vi "_Switch Polarity.vi"(0 "Lenses":T1[](array[typedef]), 1 "Start Value":dbl, 2 "Stop Value":dbl, 3 "index":i32, 4 "Unit":bool) -> (5 "Lenses 2":T1[](array[typedef]), 6 "Start Value 2":dbl, 7 "Stop Value 2":dbl)   [LabVIEW 2012]
uses:
  Type/_Lens Property.ctl
  _Global Configuration.vi
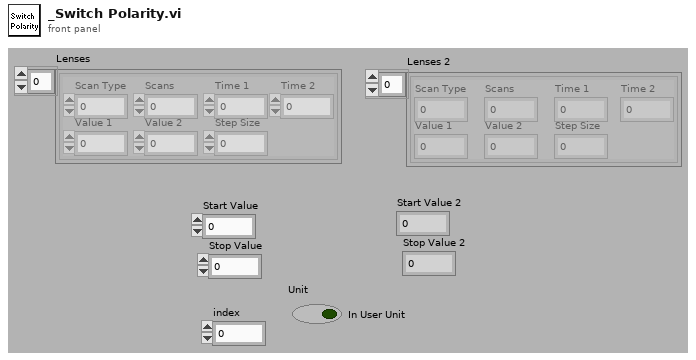
[diagram p1: front panel]
types:
  T1 = typedef "_Lens Property.ctl" = cluster{"Scan Type":u8, "Scans":i32, "Time 1":dbl, "Time 2":dbl, "Value 1":dbl, "Value 2":dbl, "Step Size":dbl}
  T2 = typedef "_RT Instrument 2.ctl" = cluster{"Table":T3[], "Instrument":string[]}
  T3 = typedef "_RT Configuration 2.ctl" = cluster{"Name":string, "Ch#":u8, "Min":dbl, "Max":dbl, "Def+":dbl, "Def-":dbl, "Offset":dbl, "Slope":dbl, "Type":u8, "Description":string, "SettleT":dbl}
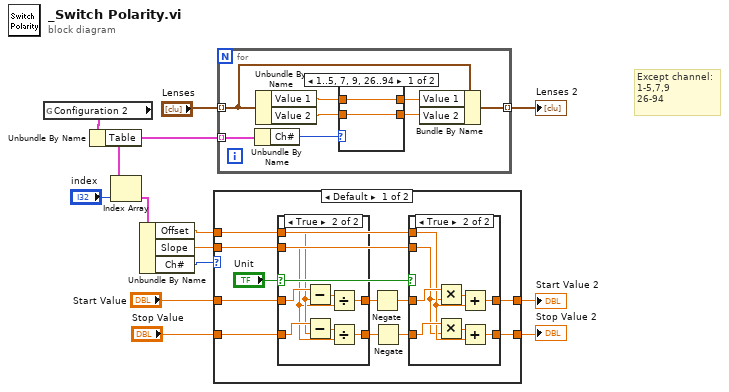
[diagram p0: block diagram]
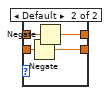
[diagram p5: hidden frame]
diagram:
  # "Except channel:\n1-5,7,9\n26-94"
  n1 = global read "_Global Configuration.vi" "Configuration 2"() -> (w5:T2)
  n2 = Unbundle By Name(w5) -> ("Table"=w3:T3[])
  n3 = Index Array(array=w3, index="index") -> (element=w1:T3)
  n4 = Unbundle By Name(w1) -> ("Offset"=w9:dbl, "Slope"=w8:dbl, "Ch#"=w7:u8)
  n5 = case shown="Default" w7 {
    tunnel: [w20 w46] -> w11
    tunnel: "Start Value" -> [w24 w46]
    tunnel: [w16 w45] -> w10
    tunnel: "Stop Value" -> [w23 w45]
    tunnel: w9 -> [w15 _]
    tunnel: w8 -> [w14 _]
    frame Default {
      n6 = case shown="True" "Unit" {
        tunnel: w15 -> [_ w40]
        tunnel: w14 -> [_ w39]
        tunnel: w24 -> [w36 w42]
        tunnel: w23 -> [w35 w41]
        tunnel: [w36 w38] -> w22
        tunnel: [w35 w37] -> w21
        frame False {
        }
        frame True {
          n7 = Subtract(x=w42, y=w40) -> (x-y=w43:dbl)
          n8 = Subtract(x=w41, y=w40) -> (x-y=w44:dbl)
          n9 = Divide(x=w43, y=w39) -> (x/y=w38:dbl)
          n10 = Divide(x=w44, y=w39) -> (x/y=w37:dbl)
        }
      }
      n11 = Negate(x=w22) -> (-x=w18:dbl)
      n12 = Negate(x=w21) -> (-x=w17:dbl)
      n13 = case shown="True" "Unit" {
        tunnel: w15 -> [_ w28]
        tunnel: w14 -> [_ w27]
        tunnel: w18 -> [w26 w32]
        tunnel: w17 -> [w25 w31]
        tunnel: [w26 w30] -> w20
        tunnel: [w25 w29] -> w16
        frame False {
        }
        frame True {
          n14 = Multiply(x=w32, y=w27) -> (x*y=w33:dbl)
          n15 = Multiply(x=w31, y=w27) -> (x*y=w34:dbl)
          n16 = Add(x=w33, y=w28) -> (x+y=w30:dbl)
          n17 = Add(x=w34, y=w28) -> (x+y=w29:dbl)
        }
      }
    }
    frame 1..5, 7, 9, 26..94 {
    }
  }
  "Stop Value 2" <- w10
  "Start Value 2" <- w11
  n18 = for {
    tunnel: "Lenses" -> [w50] mode=indexing
    tunnel: [w47] -> w4 mode=indexing
    tunnel: w3 -> [w49] mode=indexing
    n19 = Unbundle By Name(w49) -> ("Ch#"=w48:u8)
    n20 = Unbundle By Name(w50) -> ("Value 1"=w54:dbl, "Value 2"=w53:dbl)
    n21 = case shown="1..5, 7, 9, 26..94" w48 {
      tunnel: [w56 w58] -> w52
      tunnel: w54 -> [w56 w60]
      tunnel: [w55 w57] -> w51
      tunnel: w53 -> [w55 w59]
      frame 1..5, 7, 9, 26..94 {
      }
      frame Default {
        n22 = Negate(x=w59) -> (-x=w57:dbl)
        n23 = Negate(x=w60) -> (-x=w58:dbl)
      }
    }
    n24 = Bundle By Name(cluster=w50, "Value 1"=w52, "Value 2"=w51) -> (w47:T1)
  }
  "Lenses 2" <- w4
